vi "XY Graph Insert Plot.vi"(5 "Hide All Other Plots (F)":bool, 6 "Expand Legend (T)":bool=TRUE, 7 "New Plot Name (Unchanged: \"\")":string, 8 "Error In":errorcluster, 9 "Plot Index (Default Inf: Append to End)":i32=2147483647, 10 "New Plot":T1, 11 "Multiplot XY Graph Refnum in":refnum<vi>) -> (0 "Error Out":errorcluster, 2 "Plot Name":string, 3 "Multiplot XY Graph Refnum out":refnum<vi>)   [LabVIEW 2021, in "XY Graph Add-Ons.lvlib"]
doc: "Append a new plot or replace an existing plot in an existing XY Graph\n\nPlot Index = 2^21 - 1 (or Inf) --> Append\nPlot Index < 0: count plot index from end (-1: last plot, etc.)"
uses:
  XY Graph Add-Ons.lvlib
  XY Plot Data.ctl
  Graphs.lvlib
  Strings/Strings.lvlib
  Error/Error.lvlib
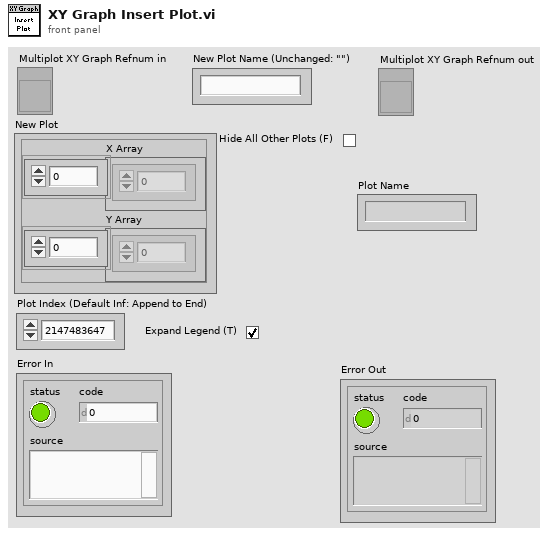
[diagram p1: front panel]
types:
  T1 = typedef "XY Graph Add-Ons.lvlib/XY Plot Data.ctl" = cluster{"X Array":dbl[], "Y Array":dbl[]}
  T2 = typedef "XY Graph Add-Ons.lvlib/XY Graph Refnum.ctl" = refnum<vi>
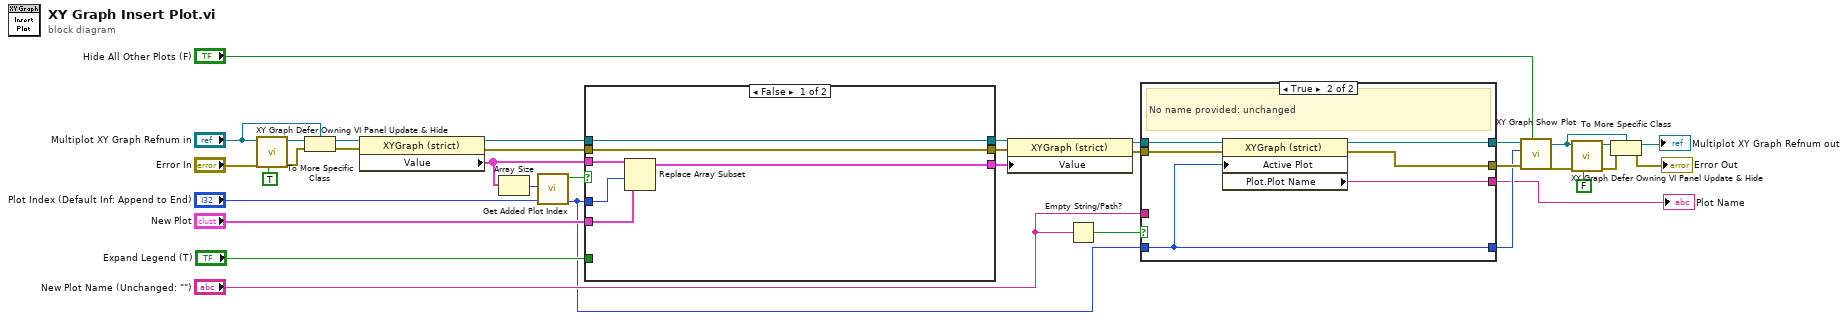
[diagram p0: block diagram]
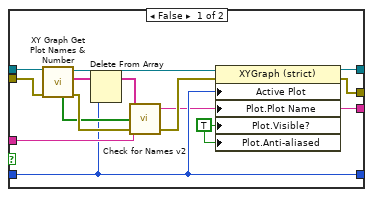
[diagram p2: hidden frame]
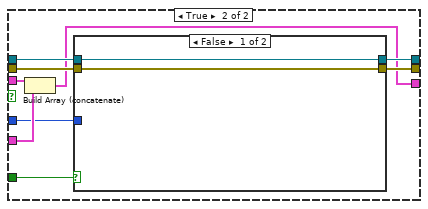
[diagram p3: hidden frame]
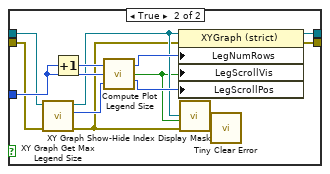
[diagram p4: hidden frame]
diagram:
  n1 = call "XY Graph Defer Owning VI Panel Update & Hide.vi"("Defer Owning Panel Update"=TRUE, "error in (no error)"="Error In", "XY Graph Refnum in"="Multiplot XY Graph Refnum in") -> ("error out"=w11:errorcluster, "XY Graph Refnum out"=w16:refnum<vi>)  [unwired: 7 in]
  n2 = To More Specific Class(target class="Multiplot XY Graph Refnum in", reference=w16, error in=w11) -> (specific class reference=w13:refnum<vi>, error out=w10:errorcluster)
  n3 = property class="XYGraph (strict)"(reference=w13, error in=w10) -> (reference out=w34:refnum<vi>, error out=w31:errorcluster, "Value"=w29:cluster{"X Array":dbl[], "Y Array":dbl[]}[])
  n4 = Array Size(array=w29) -> (size(s)=w24:i32)
  n5 = call "Get Added Plot Index.vi"("Plot Index (Append)"="Plot Index (Default Inf: Append to End)", "Graph # Plots"=w24) -> ("Actual Plot Index"=w4:i32, "Append to End?"=w26:bool)  [unwired: 8 in]
  n6 = case shown="False" w26 {
    tunnel: w29 -> [w41 w50]
    tunnel: "New Plot" -> [w40 w49]
    tunnel: [w39 w43] -> w21
    tunnel: w34 -> [w38 w47]
    tunnel: "Expand Legend (T)" -> [_ w48]
    tunnel: [w38 w46] -> w32
    tunnel: w31 -> [w37 w45]
    tunnel: [w37 w44] -> w30
    tunnel: w4 -> [w36 w42]
    frame False {
      n7 = Replace Array Subset(array=w41, new element=w40, index=w36) -> (w39:cluster{"X Array":dbl[], "Y Array":dbl[]}[])
    }
    frame True {
      n8 = Build Array (concatenate)(w50, w49) -> (w43:T1[])
      n9 = case shown="False" w48 {
        tunnel: w47 -> [w52 w57]
        tunnel: [w52 w65] -> w46
        tunnel: w45 -> [w51 w58]
        tunnel: [w51 w64] -> w44
        tunnel: w42 -> [_ w63]
        frame False {
        }
        frame True {
          n10 = call "XY Graph Get Max Legend Size.vi"("Error In"=w58, "XYGraph Refnum"=w57) -> ("Error Out"=w53:errorcluster, "Max Legend Size"=w59:i32, "XYGraph Refnum"=w55:T2)  [unwired: 6 in, 1 out]
          n11 = Increment(x=w63) -> (x+1=w62:i32)
          n12 = call "Compute Plot Legend Size.vi"("# Plots"=w62, "Current Plot (Last)"=w63, "Max Legend Size"=w59) -> ("LegNumRows"=w60:u32, "LegScrollVis"=w54:bool, "LegScrollPos"=w61:u32)  [unwired: 10 in]
          n13 = property class="XYGraph (strict)"(reference=w55, error in=w53, "LegNumRows"=w60, "LegScrollVis"=w54, "LegScrollPos"=w61) -> (reference out=w65:T2, error out=w64:errorcluster)
          n14 = call "XY Graph Show-Hide Index Display Mask.vi"("error in (no error)"=w53, "Show(T)/Hide(F)"=w54, "XYGraph Ref"=w55) -> ("error out"=w56:errorcluster)  [unwired: 7 in, 1 out]
          n15 = call "Tiny Clear Error.vi"("Error In"=w56) -> ()  [unwired: 8 in, 1 out]
        }
      }
    }
  }
  n16 = property class="XYGraph (strict)"(reference=w32, error in=w30, "Value"=w21) -> (reference out=w20:T2, error out=w19:errorcluster)
  n17 = Empty String/Path?(string/path="New Plot Name (Unchanged: \"\")") -> (empty?=w28:bool)
  n18 = case shown="True" w28 {
    tunnel: w20 -> [w75 w85]
    tunnel: [w79 w82] -> w23
    tunnel: w19 -> [w73 w84]
    tunnel: [w78 w83] -> w22
    tunnel: "New Plot Name (Unchanged: \"\")" -> [w76 _]
    tunnel: w4 -> [w67 w81]
    tunnel: [w67 w81] -> w2
    tunnel: [w66 w80] -> w1
    frame False {
      w77 = TRUE ("Plot.Visible")
      n19 = call "XY Graph Get Plot Names & Number.vi"("error in (no error)"=w73, "XYGraph in"=w75) -> ("error out"=w72:errorcluster, "Plot Names"=w70:string[], "XYGraph out"=w74:T2, "Empty Plots?"=w68:bool[])  [unwired: 4 in, 2 out]
      n20 = Delete From Array(array=w70, index=w67) -> (array with subset deleted=w69:string[])  [unwired: 1 in, 1 out]
      n21 = call "Check for Names v2.vi"("New Name"=w76, "Name List"=w69, "Empty Plots?"=w68, "Error In"=w72) -> ("New Name"=w66:string, "Error Out"=w71:errorcluster)  [unwired: 2 in, 2 out]
      n22 = property class="XYGraph (strict)"(reference=w74, error in=w71, "Active Plot"=w67, "Plot.Plot Name"=w66, "Plot.Visible?"=w77, "Plot.Anti-aliased"=w77) -> (reference out=w79:T2, error out=w78:errorcluster)
    }
    frame True {
      # "No name provided: unchanged"
      n23 = property class="XYGraph (strict)"(reference=w85, error in=w84, "Active Plot"=w81) -> (reference out=w82:T2, error out=w83:errorcluster, "Plot.Plot Name"=w80:string)
    }
  }
  "Plot Name" <- w1
  n24 = call "XY Graph Show Plot.vi"("Hide All Other Plots (F)"="Hide All Other Plots (F)", "error in (no error)"=w22, "Selected Plot Index"=w2, "XYGraph in"=w23) -> ("error out"=w18:errorcluster, "XYGraph out"=w7:T2)  [unwired: 6 in]
  n25 = call "XY Graph Defer Owning VI Panel Update & Hide.vi"("Defer Owning Panel Update"=FALSE, "error in (no error)"=w18, "XY Graph Refnum in"=w7) -> ("error out"=w6:errorcluster, "XY Graph Refnum out"=w9:refnum<vi>)  [unwired: 7 in]
  n26 = To More Specific Class(target class=w7, reference=w9, error in=w6) -> (specific class reference=→"Multiplot XY Graph Refnum out":T2, error out=→"Error Out":errorcluster)
